vi "Set_Freq_Table.vi"(4 "error in (no error)":errorcluster, 6 "step(Mhz)":dbl, 7 "freq_min(Mhz)":dbl) -> (0 "error out":errorcluster, 2 "freq_table":dbl[](array[numeric]), 3 "Count":dbl)   [LabVIEW 2015]
panel:
  in  "freq_max(Mhz)":dbl
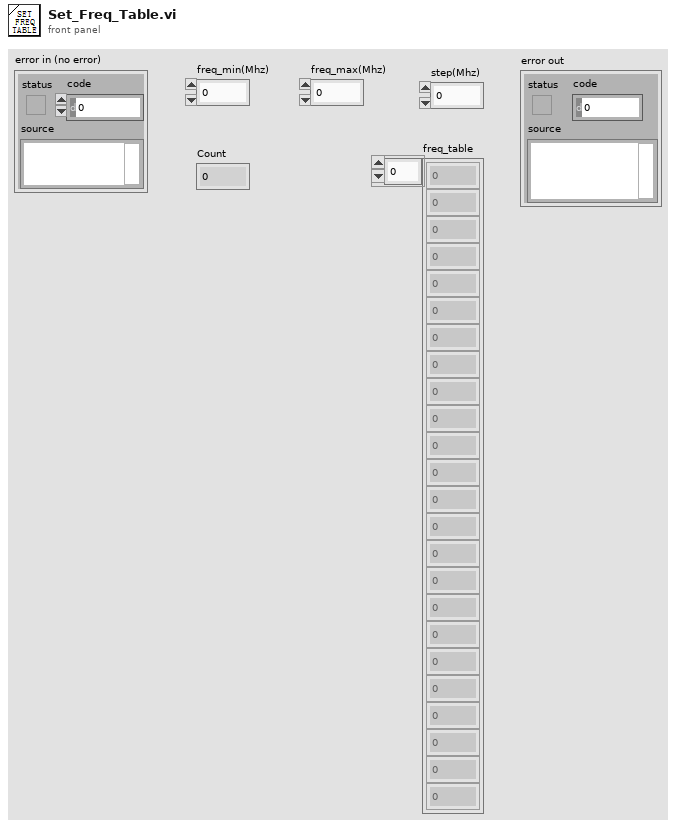
[diagram p1: front panel]
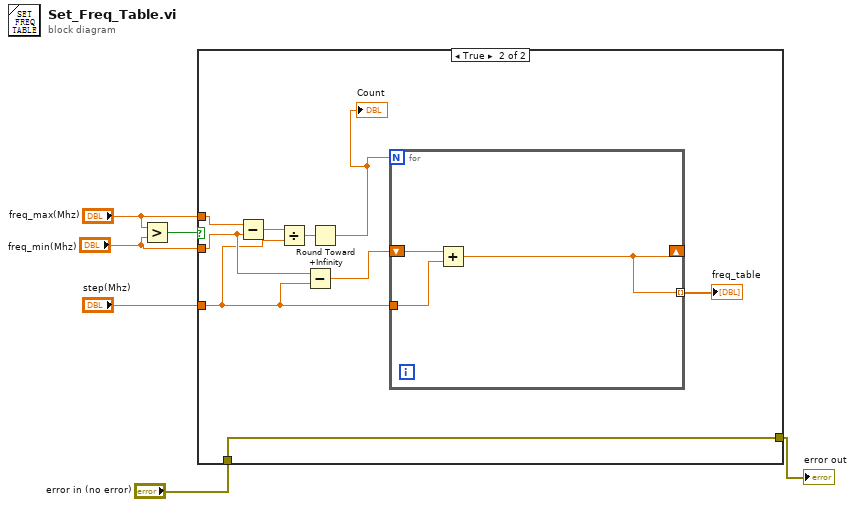
[diagram p0: block diagram]
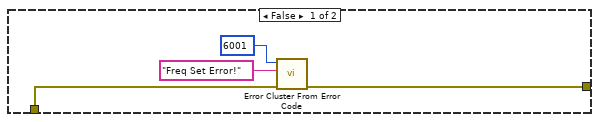
[diagram p2: hidden frame]
diagram:
  n1 = Greater?(x="freq_max(Mhz)", y="freq_min(Mhz)") -> (0:w6:bool)
  n2 = case shown="True" w6 {
    tunnel: "error in (no error)" -> [w8 w19]
    tunnel: [w7 w19] -> w4
    tunnel: "freq_max(Mhz)" -> [_ w18]
    tunnel: "freq_min(Mhz)" -> [_ w13]
    tunnel: "step(Mhz)" -> [_ w12]
    frame False {
      n3 = call <vilib>:"Error Cluster From Error Code.vi"("error in (no error)"=w8, "error message (\"\")"="Freq Set Error!" ("error message (\"\")"), "error code (0)"=6001) -> ("error out"=w7:errorcluster)  [unwired: 6 in]
    }
    frame True {
      n4 = Subtract(x=w18, y=w13) -> (x-y=w17:dbl)
      n5 = Divide(x=w17, y=w12) -> (x/y=w16:dbl)
      n6 = Subtract(x=w13, y=w12) -> (x-y=w11:dbl)
      n7 = Round Toward +Infinity(x=w16) -> (ceil(x): smallest int >= x=w15:dbl)
      "Count" <- w15
      n8 = for {
        N: w15 -> [_]
        shift-right: [w20] -> _
        shift-left: w11 -> [w22]
        tunnel: w12 -> [w21]
        tunnel: [w20] -> w14 mode=indexing
        n9 = Add(x=w22, y=w21) -> (x+y=w20:dbl)
      }
      "freq_table" <- w14
    }
  }
  "error out" <- w4
